vi "Decode JWT Header.vi"(0 "JSONWebToken in":refnum<class "JSONWebToken.lvclass">, 11 "error in (no error)":errorcluster) -> (3 "header (JSON)":string, 4 "JSONWebToken out":refnum<class "JSONWebToken.lvclass">, 6 "JWT header":T1, 15 "error out":errorcluster)   [LabVIEW 2017, in "JSONWebToken.lvclass"]
doc: "<B>JOSE Header</B>\n\n For a JWT object, the members of the JSON object represented by the JOSE Header describe the cryptographic operations applied to the JWT and optionally, additional properties of the JWT."
uses:
  JSONWebToken.lvclass
  header.ctl
  JSONWebToken.lvclass/JSONWebToken.ctl
  40378a84-5f64-4a5f-a7f2-21a6353c70a4.vi
  <vilib>/addons/_JKI.lib/Serialization/JSON/JKI JSON Serialization.lvlib
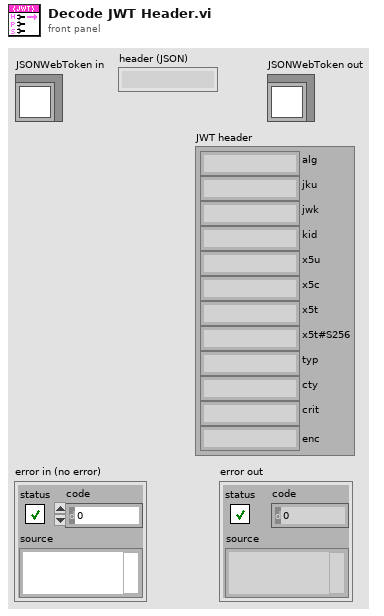
[diagram p1: front panel]
types:
  T1 = typedef "JSONWebToken.lvclass/header.ctl" = cluster{"alg":string, "jku":string, "jwk":string, "kid":string, "x5u":string, "x5c":string, "x5t":string, "x5t#S256":string, "typ":string, "cty":string, "crit":string, "enc":string}
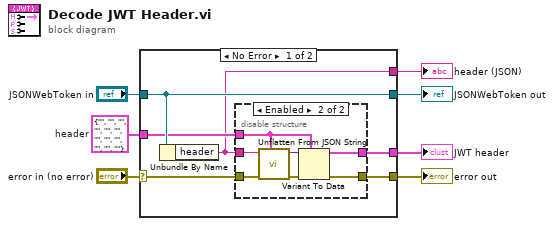
[diagram p0: block diagram]
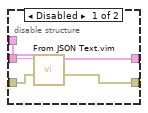
[diagram p2: hidden frame]
diagram:
  w3 = T1 {"alg"="", "jku"="", "jwk"="", "kid"="", "x5u"="", "x5c"="", "x5t"="", "x5t#S256"="", "typ"="", "cty"="", "crit"="", "enc"=""}  # header
  n1 = case shown="No Error" "error in (no error)" {
    selector: "error in (no error)" -> [w11 w28]
    tunnel: [w10 w28] -> w6
    tunnel: [w13 w27] -> w4
    tunnel: "JSONWebToken in" -> [w13 w27]
    tunnel: w3 -> [w12 w26]
    tunnel: [w9 w26] -> w2
    tunnel: [w8 _] -> w1
    frame No Error {
      n2 = Unbundle By Name(w13) -> ("header"=w8:string)
      n3 = disable-structure shown="Enabled" {
        disable-tunnel: w8 -> [w18 w25]
        disable-tunnel: w12 -> [w17 w21]
        disable-tunnel: w11 -> [w16 w24]
        disable-tunnel: [w15 w19] -> w10
        disable-tunnel: [w14 w20] -> w9
        frame Disabled {
          n4 = call "From JSON Text.vim"("Data Type and Default Value"=w17, "error in (no error)"=w16, "JSON"=w18) -> ("error out"=w15:errorcluster, "Data out"=w14:T1)  [unwired: 7 in]
        }
        frame Enabled {
          n5 = call <vilib>:"Unflatten From JSON String.vi"("Type and Defaults"=w21, "error in"=w24, "JSON String"=w25) -> ("error out"=w23:errorcluster, "Variant"=w22:variant)  [unwired: 7 in]
          n6 = Variant To Data(error in=w23, type=w21, Variant=w22) -> (data=w20:T1, error out=w19:errorcluster)
        }
      }
    }
    frame Error {
    }
  }
  "error out" <- w6
  "JSONWebToken out" <- w4
  "JWT header" <- w2
  "header (JSON)" <- w1
